vi "Move.vi"(0 "ASI stage":T1, 1 "Axis configuration":u16(ring)=5 items=["No axis", "X", "Y", "Z", "XY", "XYZ"], 5 "x":dbl, 7 "y":dbl, 9 "z":dbl, 11 "error in (no error)":errorcluster) -> (4 "ASI stage out":T1, 15 "error out":errorcluster)   [LabVIEW 2010]
uses:
  stage properties.ctl
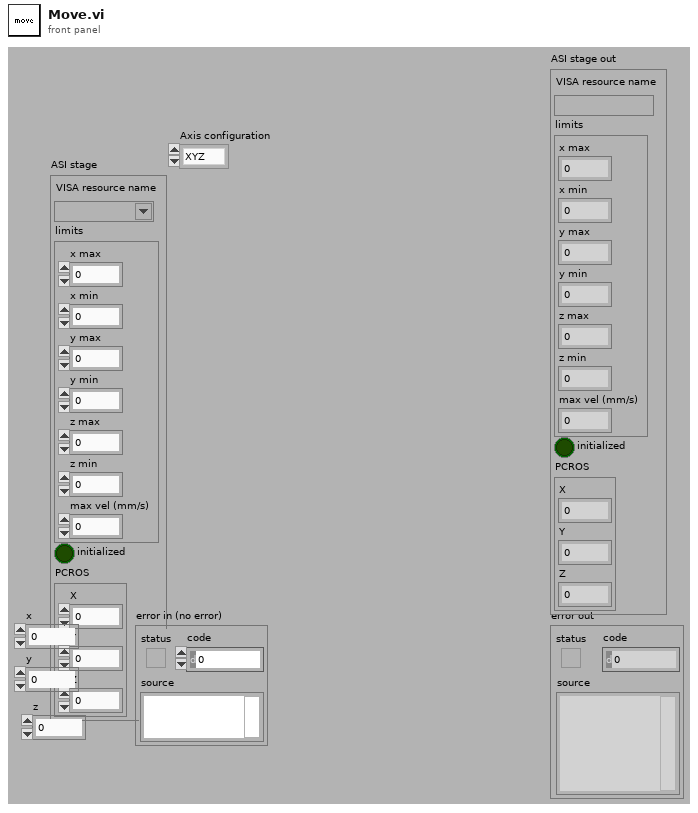
[diagram p1: front panel]
types:
  T1 = typedef "stage properties.ctl" = cluster{"VISA resource name":refnum<visa-resource-name>, "limits":cluster{"x max":dbl, "x min":dbl, "y max":dbl, "y min":dbl, "z max":dbl, "z min":dbl, "max vel (mm/s)":dbl}, "initialized":bool, "PCROS":cluster{"X":dbl, "Y":dbl, "Z":dbl}}
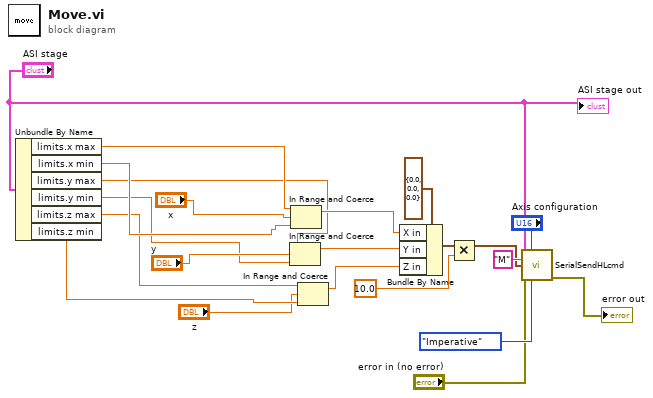
[diagram p0: block diagram]
diagram:
  n1 = Unbundle By Name("ASI stage") -> ("limits.x max"=w17:dbl, "limits.x min"=w10:dbl, "limits.y max"=w9:dbl, "limits.y min"=w8:dbl, "limits.z max"=w7:dbl, "limits.z min"=w6:dbl)
  n2 = In Range and Coerce(upper limit=w9, x="y", lower limit=w8) -> (coerced(x)=w14:dbl)  [unwired: 1 out]
  n3 = In Range and Coerce(upper limit=w17, x="x", lower limit=w10) -> (coerced(x)=w13:dbl)  [unwired: 1 out]
  n4 = In Range and Coerce(upper limit=w7, x="z", lower limit=w6) -> (coerced(x)=w4:dbl)  [unwired: 1 out]
  n5 = Bundle By Name(cluster=cluster{"X in":dbl, "Y in":dbl, "Z in":dbl} {"X in"=0.0, "Y in"=0.0, "Z in"=0.0} ("data in"), "X in"=w13, "Y in"=w14, "Z in"=w4) -> (w12:cluster{"X in":dbl, "Y in":dbl, "Z in":dbl})
  n6 = Multiply(x=w12, y=10.0 ("z")) -> (x*y=w2:cluster{"X in":dbl, "Y in":dbl, "Z in":dbl})
  n7 = call "SerialSendHLcmd.vi"("ASI stage"="ASI stage", "Axis configuration"="Axis configuration", "Command"="M", "data in"=w2, "error in (no error)"="error in (no error)", "Command type"=enum16{"Query", "Where", "Imperative", "DU Y"}."Imperative") -> ("error out"=→"error out":errorcluster)  [unwired: 7 in, 2 out]
  "ASI stage out" <- "ASI stage"
